vi "Xml_Create_Default.vi"(8 "error in (no error)":errorcluster) -> (0 "error out":errorcluster)   [LabVIEW 2018]
doc: "This example demonstrates how to convert a LabVIEW data structure into an XML string using the GXML reference library."
uses:
  controls/TRAPPING_Inputs.ctl
  controls/SPECTRUM.ctl
  controls/VOLTAGES_Inputs.ctl
  controls/HEXA_Inputs.ctl
  controls/QUAD_Inputs.ctl
  controls/DATA_Inputs.ctl
  controls/PROCESSING_Inputs.ctl
  controls/HARDWARE_Inputs.ctl
  controls/AO_6711_Inputs.ctl
  controls/AWG_5421_Inputs.ctl
  <instrlib>/niFgen/niFgen.llb/niFgen_ctl Trigger Source Values (Ring).ctl
  controls/DIGIT_5122_Inputs.ctl
  <instrlib>/niScope/Controls/niScope trigger source.ctl
  controls/HSDIO_6541_Inputs.ctl
  <instrlib>/niHSDIO/niHSDIO.llb/niHSDIO_ctl Trigger Source Values (Ring).ctl
  controls/EXPERT_Inputs.ctl
  controls/SOFTWARE_Inputs.ctl
  controls/XML_Inputs.ctl
  controls/TIMING_Inputs.ctl
  controls/EXCIT_Table.ctl
  controls/EXCIT_Inputs.ctl
  controls/EXPERT_Path_Selector.ctl
  <vilib>/NI/GXML/GXML.lvlib
panel:
  out "chemin complet":path
  in  "EXCIT Table":T1={"Number of Excits"=0, "Number of Ejects"=0, "Sampling Frequency"=0.0, "Waveforms Table"=[["Excit1", "name", "Swift", "0.5", "1200", "70", "150", "550", "0", "0", "0"]]}
  in  "SOFTWARE Inputs":T2={"Application Directory"=path "D:/S.O.F.T.S/LABVIEW/PIL", "Software Version"="1.0.0", "Data Path"=path "D:/PIRENEA/DATA", "XML Path"=path "D:/PIRENEA/DATA", "XML File Filter"="*.xml", "XML Saved Path"=path "D:/PIRENEA/SAVED_XML", "Excit Scripts Path"=path "D:/PIRENEA/TECHNICAL/EXCIT_SCRIPTS", "Excit Scripts File Filter"="*.txt", "Excit Waveforms Path"=path "D:/PIRENEA/TECHNICAL/EXCIT_WFMS", "Excit Waveforms File Filter"="*.bin", "Timing Scripts Path"=path "D:/PIRENEA/TECHNICAL/TIMING_SCRIPTS", "Timing Scripts File Filter"="*.txt", "Timing Waveforms Path"=path "D:/PIRENEA/TECHNICAL/TIMING_WFMS", "Timing Waveforms File Filter"="*.bin", "Trapping Waveforms Path"=path "D:/PIRENEA/TECHNICAL/TRAPPING_WFMS", "Trapping Waveforms File Filter"="*.bin"}
  in  "TIMING Inputs":T3={"Number of Acquisitions "=1, "Number of Accumulations"=1, "Table of Waveforms"=[], "Script Text"=""} caption="SEQUENCE Inputs" {"Number of Accumulations" min=0 max=50 step=1; "Number of Acquisitions" min=1 max=10 step=1}
  in  "EXPERT Inputs":T4={"DIGIT 5122 Inputs"={"Sample Rate"=10000.0, "Resource Name"="DIGIT_5122", "Channel Name"="0", "Trigger Source"="VAL_EXTERNAL", "Vertical Range"=10.0, "Trigger Level"=3.0}, "HSDIO 6541 Inputs"={"Resource Name"="HSDIO_6541", "Clock Rate"=1000000.0, "Trigger Source"="PFI0"}, "SOFTWARE Inputs"={"Application Directory"=path "D:/S.O.F.T.S/LABVIEW/PIL", "Software Version"="1.0.0", "Data Path"=path "D:/PIRENEA/DATA", "XML Path"=path "D:/PIRENEA/DATA", "XML File Filter"="*.xml", "XML Saved Path"=path "D:/PIRENEA/DATA", "Excit Scripts Path"=path "D:/PIRENEA/EXCIT_SCRIPTS", "Excit Scripts File Filter"="*.txt", "Excit Waveforms Path"=path "D:/PIRENEA/EXCIT_WFMS", "Excit Waveforms File Filter"="*.bin", "Timing Scripts Path"=path "D:/PIRENEA/SEQUENCE_SCRIPTS", "Timing Scripts File Filter"="*.txt", "Timing Waveforms Path"=path "D:/PIRENEA/SEQUENCE_WFMS", "Timing Waveforms File Filter"="*.bin", "Trapping Waveforms Path"=path "D:/PIRENEA/TRAPPING_WFMS", "Trapping Waveforms File Filter"="*.bin"}, "AO 6711 Inputs"={"Physical Channels"="AO_6711/ao0:3", "Min Voltage"=-10.0, "Max Voltage"=10.0, "Trigger Source"="/AO_6711/PFI0", "Counter"="AO_6711/ctr0"}, "AWG 5421 Inputs"={"Resource Name"="AWG_5421", "Sample Rate"=20000000.0, "Trigger Type"=2, "Trigger Source"="PFI0", "Waveform Gain"=0.31, "Digital Filter ON"=TRUE}, "XML Inputs"={"Version Tag Name"="XML_Version", "Version String"="1.0"}} {"AWG 5421 Inputs"."Sample Rate" format="%.2p"; "AWG 5421 Inputs"."Trigger Type" items=["None", "Software Edge", "Digital Edge", "Digital Level"]; "AO 6711 Inputs"."Max Voltage" min=-10.0 max=10.0; "AO 6711 Inputs"."Min Voltage" min=-10.0 max=10.0; "HSDIO 6541 Inputs"."Clock Rate" format="%.2p"; "DIGIT 5122 Inputs"."Trigger Level" format="%.2f"; "DIGIT 5122 Inputs"."Vertical Range" format="%.2f"; "DIGIT 5122 Inputs"."Sample Rate" step=65535.0 format="%#_3p"}
  in  "HARDWARE Inputs":T13={"AO 6711 Inputs"={"Physical Channels"="AO_6711/ao0:3", "Min Voltage"=-10.0, "Max Voltage"=10.0, "Trigger Source"="/AO_6711/PFI3", "Counter"="AO_6711/ctr0"}, "AWG 5421 Inputs"={"Resource Name"="AWG_5421", "Sample Rate"=10000000.0, "Trigger Type"=2, "Trigger Source"="PFI0", "Waveform Gain"=0.31, "Digital Filter ON"=TRUE}, "DIGIT 5122 Inputs"={"Sample Rate"=10000.0, "Resource Name"="DIGIT_5122", "Channel Name"="0", "Trigger Source"="VAL_EXTERNAL", "Vertical Range"=10.0, "Trigger Level"=3.0}, "HSDIO 6541 Inputs"={"Resource Name"="HSDIO_6541", "Clock Rate"=1000000.0, "Trigger Source"="PFI0"}} {"HSDIO 6541 Inputs"."Clock Rate" format="%.2p"; "DIGIT 5122 Inputs"."Trigger Level" format="%.2f"; "DIGIT 5122 Inputs"."Vertical Range" format="%.2f"; "DIGIT 5122 Inputs"."Sample Rate" step=65535.0 format="%#_3p"; "AWG 5421 Inputs"."Sample Rate" format="%.2p"; "AWG 5421 Inputs"."Trigger Type" items=["None", "Software Edge", "Digital Edge", "Digital Level"]; "AO 6711 Inputs"."Max Voltage" min=-10.0 max=10.0; "AO 6711 Inputs"."Min Voltage" min=-10.0 max=10.0}
  in  "PROCESSING Inputs":T14={"Reference Mass"=300.0939, "Cyclotron Freq"=255.727, "Magnetron Freq"=0.001} {"Magnetron Freq" format="%.5g"; "Cyclotron Freq" format="%.5g"; "Reference Mass" format="%.5g"}
  in  "DATA Inputs":T15={"Record Length"=100000, "Sample Rate"=10000000.0, "Data Type"=0, "Vertical Range"=0.4, "Acquisition Duration"=100000.0} {"Vertical Range" items=["0.2"=0.2, "0.4"=0.4, "1"=1.0, "2"=2.0, "4"=4.0, "10"=10.0]; "Data Type" items=["I16", "DBL"]; "Sample Rate" items=["1 MHz"=1000000.0, "2 MHz"=2000000.0, "5 MHz"=5000000.0, "10 MHz"=10000000.0, "20 MHz"=20000000.0, "25 MHz"=25000000.0, "50 MHz"=50000000.0, "100 MHz"=100000000.0]}
  in  "Version String":string="1.4"
  in  "Version Tag Name":string="XML_Version"
  out "Version String":string
  in  "VOLTAGES Inputs":T16={"Hexa 1"={"Used"=TRUE, "Voltage"=0.1}, "Hexa 2"={"Used"=TRUE, "Voltage"=0.2}, "Hexa 3"={"Used"=TRUE, "Voltage"=0.3}, "Quad 1"={"Used"=TRUE, "Voltage"=1.1}, "Quad 2"={"Used"=TRUE, "Voltage"=1.2}, "Quad 3"={"Used"=TRUE, "Voltage"=1.3}}
  in  "SPECTRUM":T19={"Day Path"=path "D:/PIRENEA/DATA/2016/data_2016_01_01", "Spectrum Name"="2016_01_01_000.A00", "Accumulated"=FALSE, "Stored in Database"=FALSE, "From a Set of"=1, "Quality Flag"="Optimal"}
  in  "TRAPPING Inputs":T20={"Number of Channels"=4, "Init Values"=[2.0, 9.0, 2.0, 9.0], "Opening Values"=[0.0, 0.0, 0.0, 0.0], "Trapping Values"=[2.0, 9.0, 2.0, 9.0], "Emptying Values"=[-10.0, -10.0, -10.0, -10.0], "Adiabatic ON"=FALSE, "Adiabatic Duration"=0, "Adiabatic Waveforms"=["Adiabatic_None_2_2_2000", "Adiabatic_Ramp_9_0_2000", "Adiabatic_DoubleRamp_2_0_2000", "Adiabatic_RC_9_0_2000"], "Ions Accumulation ON"=FALSE, "Number of Ions Refills"=1, "Ions Opening Values"=[0.0, 0.0, 0.0, 0.0], "Ions Trapping Values"=[2.0, 9.0, 2.0, 9.0]} {"Number of Ions Refills" min=1 max=1000; "Ions Opening Values" min=-10.0 max=10.0; "Ions Trapping Values" min=-10.0 max=10.0; "Trapping Values" min=-10.0 max=10.0; "Init Values" min=-10.0 max=10.0; "Emptying Values" min=-10.0 max=10.0; "Opening Values" min=-10.0 max=10.0}
  in  "Save XML to File?":bool
  out "Concatenated GXML String":string
  # "HEXAPOLE"
  # "QUADRIPOLE"
  # "GO_out"
  # "Gout"
  # "GI_in"
  # "Gin"
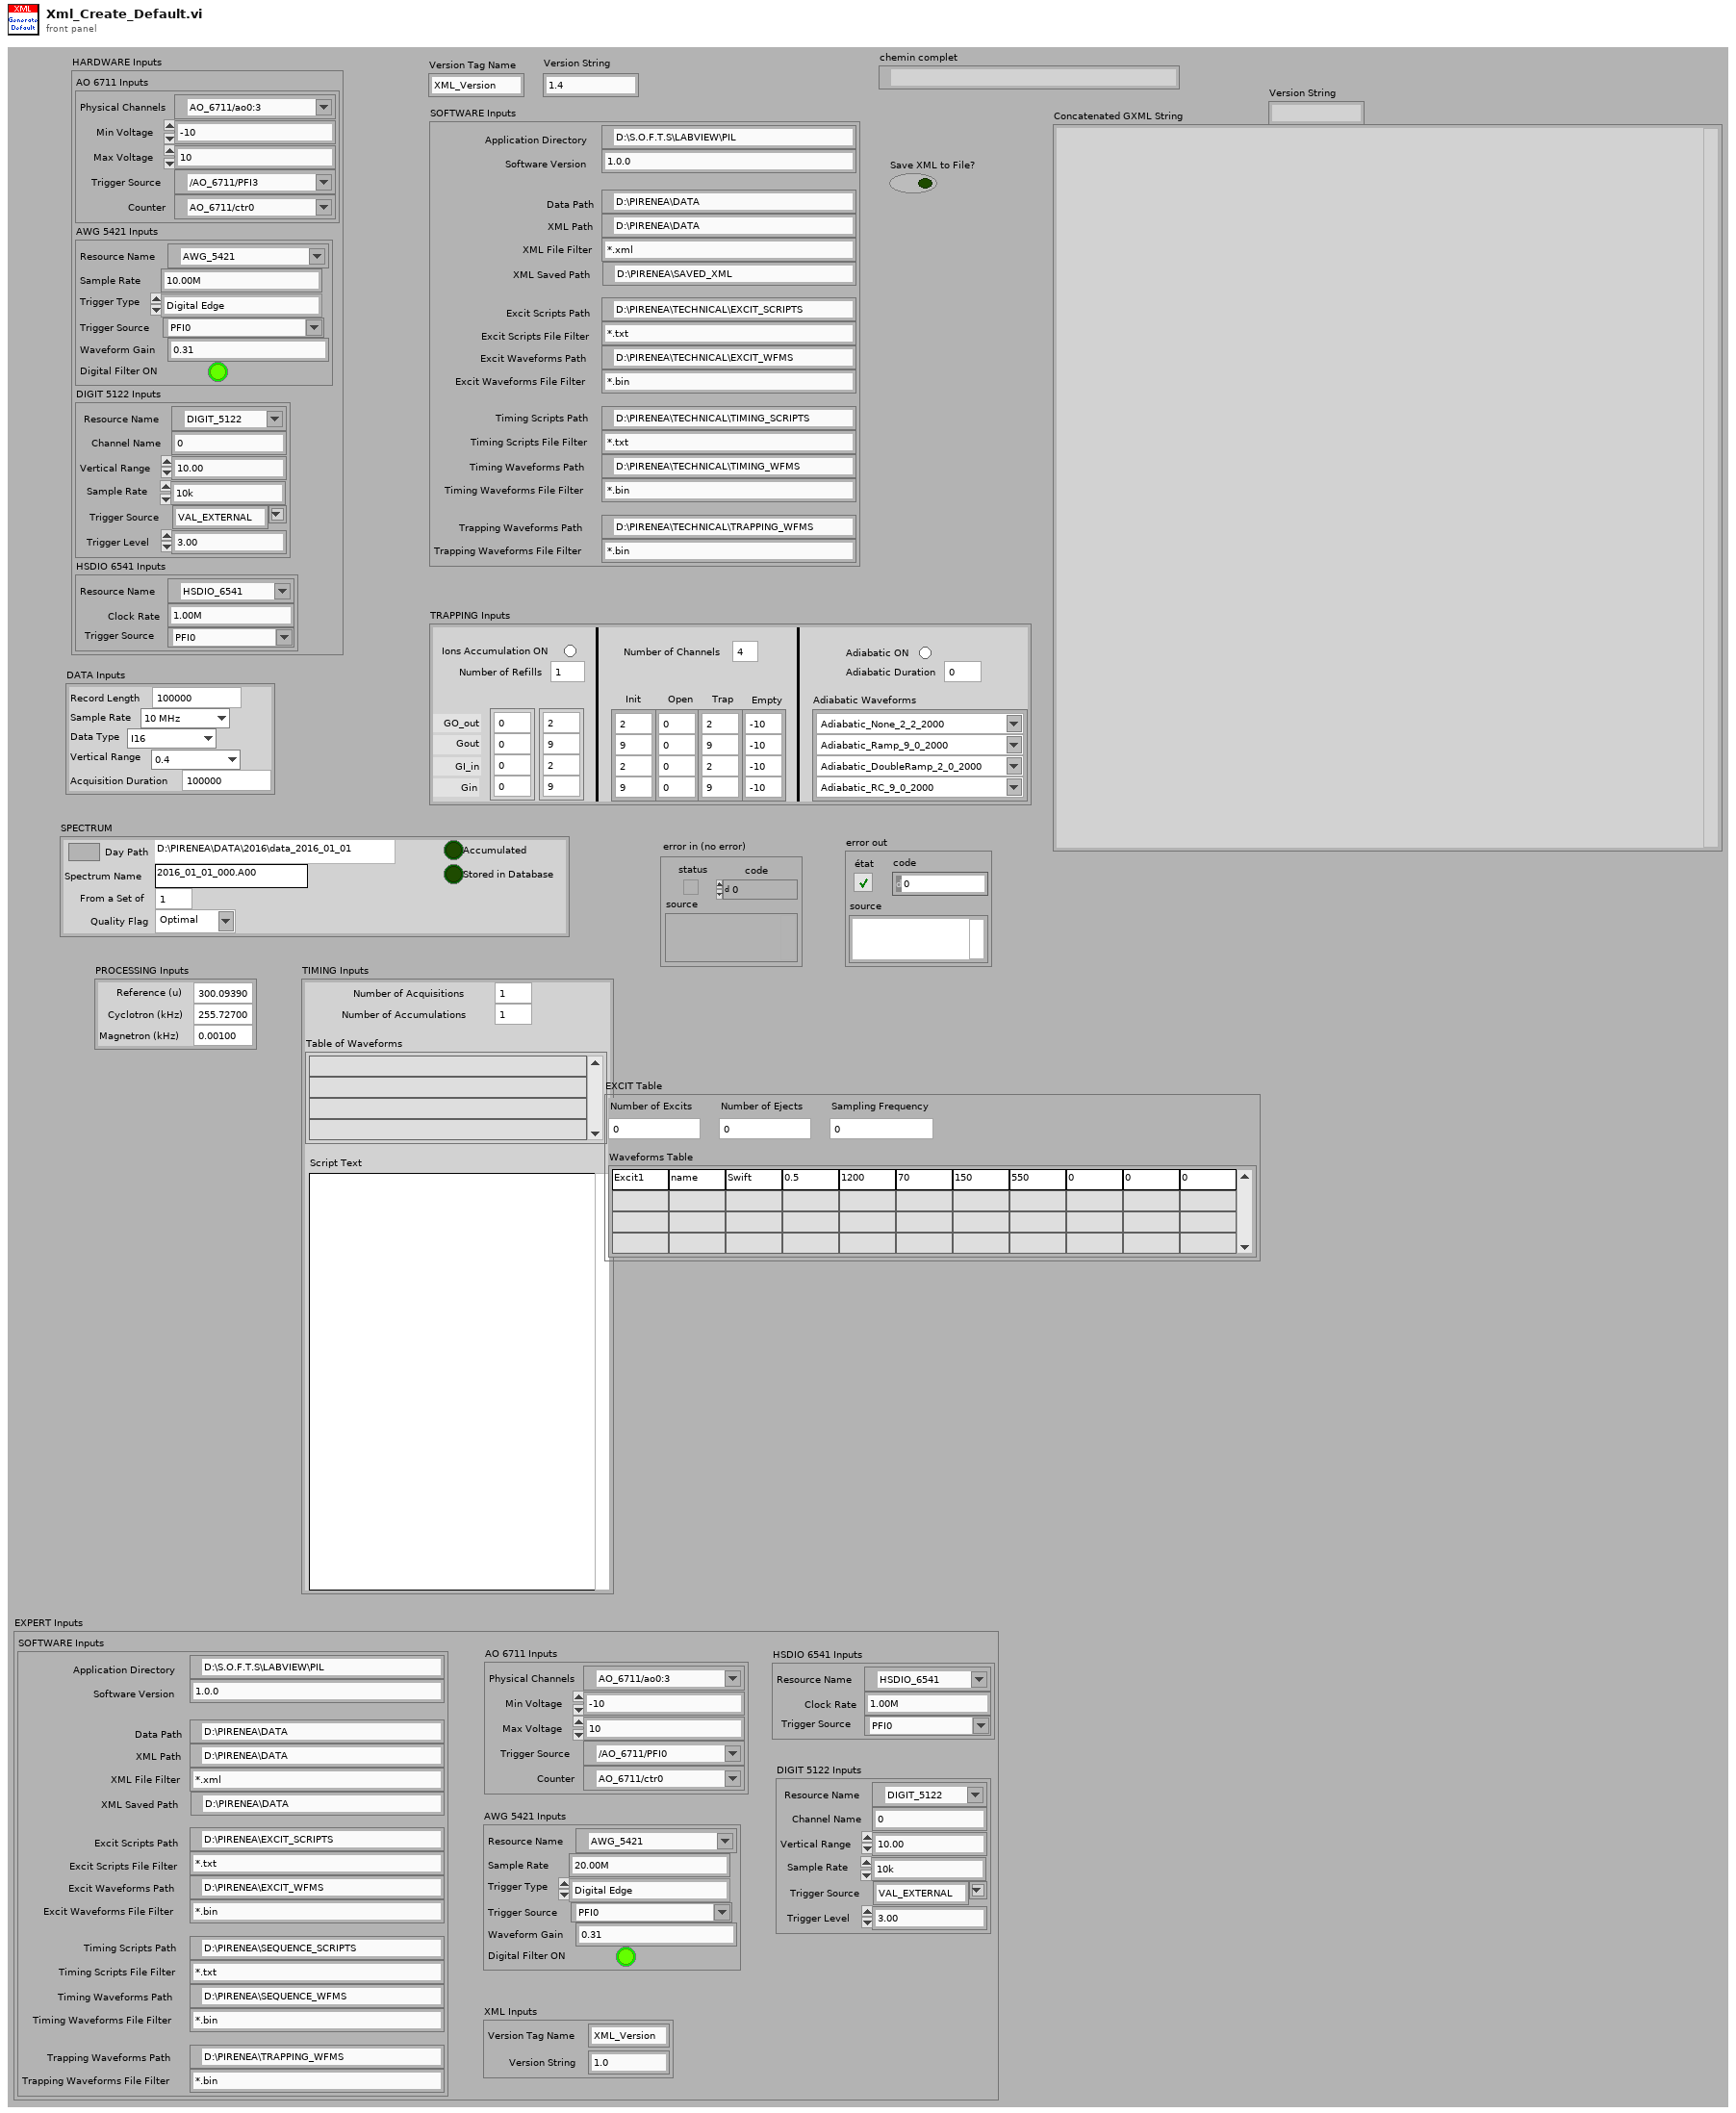
[diagram p1: front panel]
types:
  T1 = typedef "EXCIT_Table.ctl" = cluster{"Number of Excits":u16, "Number of Ejects":u16, "Sampling Frequency":dbl, "Waveforms Table":string[][]}
  T2 = typedef "SOFTWARE_Inputs.ctl" = cluster{"Application Directory":path, "Software Version":string, "Data Path":path, "XML Path":path, "XML File Filter":string, "XML Saved Path":path, "Excit Scripts Path":path, "Excit Scripts File Filter":string, "Excit Waveforms Path":path, "Excit Waveforms File Filter":string, "Timing Scripts Path":path, "Timing Scripts File Filter":string, "Timing Waveforms Path":path, "Timing Waveforms File Filter":string, "Trapping Waveforms Path":path, "Trapping Waveforms File Filter":string}
  T3 = typedef "TIMING_Inputs.ctl" = cluster{"Number of Acquisitions ":i16, "Number of Accumulations":i16, "Table of Waveforms":string[], "Script Text":string}
  T4 = typedef "EXPERT_Inputs.ctl" = cluster{"DIGIT 5122 Inputs":T5, "HSDIO 6541 Inputs":T7, "SOFTWARE Inputs":T2, "AO 6711 Inputs":T9, "AWG 5421 Inputs":T10, "XML Inputs":T12}
  T5 = typedef "DIGIT_5122_Inputs.ctl" = cluster{"Sample Rate":dbl, "Resource Name":refnum<k15>, "Channel Name":string, "Trigger Source":T6, "Vertical Range":dbl, "Trigger Level":dbl}
  T6 = typedef "niScope trigger source.ctl" = string
  T7 = typedef "HSDIO_6541_Inputs.ctl" = cluster{"Resource Name":refnum<k15>, "Clock Rate":dbl, "Trigger Source":T8}
  T8 = typedef "niHSDIO_ctl Trigger Source Values (Ring).ctl" = string
  T9 = typedef "AO_6711_Inputs.ctl" = cluster{"Physical Channels":tag, "Min Voltage":dbl, "Max Voltage":dbl, "Trigger Source":tag, "Counter":tag}
  T10 = typedef "AWG_5421_Inputs.ctl" = cluster{"Resource Name":refnum<k15>, "Sample Rate":dbl, "Trigger Type":u16, "Trigger Source":T11, "Waveform Gain":dbl, "Digital Filter ON":bool}
  T11 = typedef "niFgen_ctl Trigger Source Values (Ring).ctl" = string
  T12 = typedef "XML_Inputs.ctl" = cluster{"Version Tag Name":string, "Version String":string}
  T13 = typedef "HARDWARE_Inputs.ctl" = cluster{"AO 6711 Inputs":T9, "AWG 5421 Inputs":T10, "DIGIT 5122 Inputs":T5, "HSDIO 6541 Inputs":T7}
  T14 = typedef "PROCESSING_Inputs.ctl" = cluster{"Reference Mass":dbl, "Cyclotron Freq":dbl, "Magnetron Freq":dbl}
  T15 = typedef "DATA_Inputs.ctl" = cluster{"Record Length":i32, "Sample Rate":dbl, "Data Type":u8, "Vertical Range":dbl, "Acquisition Duration":dbl}
  T16 = typedef "VOLTAGES_Inputs.ctl" = cluster{"Hexa 1":T17, "Hexa 2":T17, "Hexa 3":T17, "Quad 1":T18, "Quad 2":T18, "Quad 3":T18}
  T17 = typedef "HEXA_Inputs.ctl" = cluster{"Used":bool, "Voltage":dbl}
  T18 = typedef "QUAD_Inputs.ctl" = cluster{"Used":bool, "Voltage":dbl}
  T19 = typedef "SPECTRUM.ctl" = cluster{"Day Path":path, "Spectrum Name":string, "Accumulated":bool, "Stored in Database":bool, "From a Set of":i16, "Quality Flag":string}
  T20 = typedef "TRAPPING_Inputs.ctl" = cluster{"Number of Channels":i32, "Init Values":dbl[], "Opening Values":dbl[], "Trapping Values":dbl[], "Emptying Values":dbl[], "Adiabatic ON":bool, "Adiabatic Duration":i32, "Adiabatic Waveforms":string[], "Ions Accumulation ON":bool, "Number of Ions Refills":i32, "Ions Opening Values":dbl[], "Ions Trapping Values":dbl[]}
  T21 = typedef "EXPERT_Path_Selector.ctl" = enum16{"Application", "Resources", "Data", "XML", "XML Saved", "Load Directory"}
  T22 = typedef "EXCIT_Inputs.ctl" = cluster{"Number of Excitations":i32, "Script Text":string, "Table of Waveforms":string[]}
  T23 = typedef "EXPERIMENT_Inputs.ctl" = cluster{"Setup":string, "Date":string, "User Name":string, "Comment":string, "Experiment Procedures":string[], "Chemical Source":string, "Sample Components":string[], "Species":string[], "Laser 1":T24, "Laser 2":T24, "Laser 3":T24, "Laser 4":T24, "Laser 5":T24, "Lamp 1":T25, "Lamp 2":T25, "Gas 1":T26, "Gas 2":T26, "Gas 3":T26, "Gas 4":T26, "Gas 5":T26}
  T24 = typedef "LASER_Inputs.ctl" = cluster{"Used":bool, "Name":string, "Wavelength":dbl, "Energy":dbl}
  T25 = typedef "LAMP_Inputs.ctl" = cluster{"Used":bool, "Name":string, "Wavelength":dbl, "Attenuation":dbl}
  T26 = typedef "GAS_Inputs.ctl" = cluster{"Used":bool, "Name":string, "Pressure":dbl}
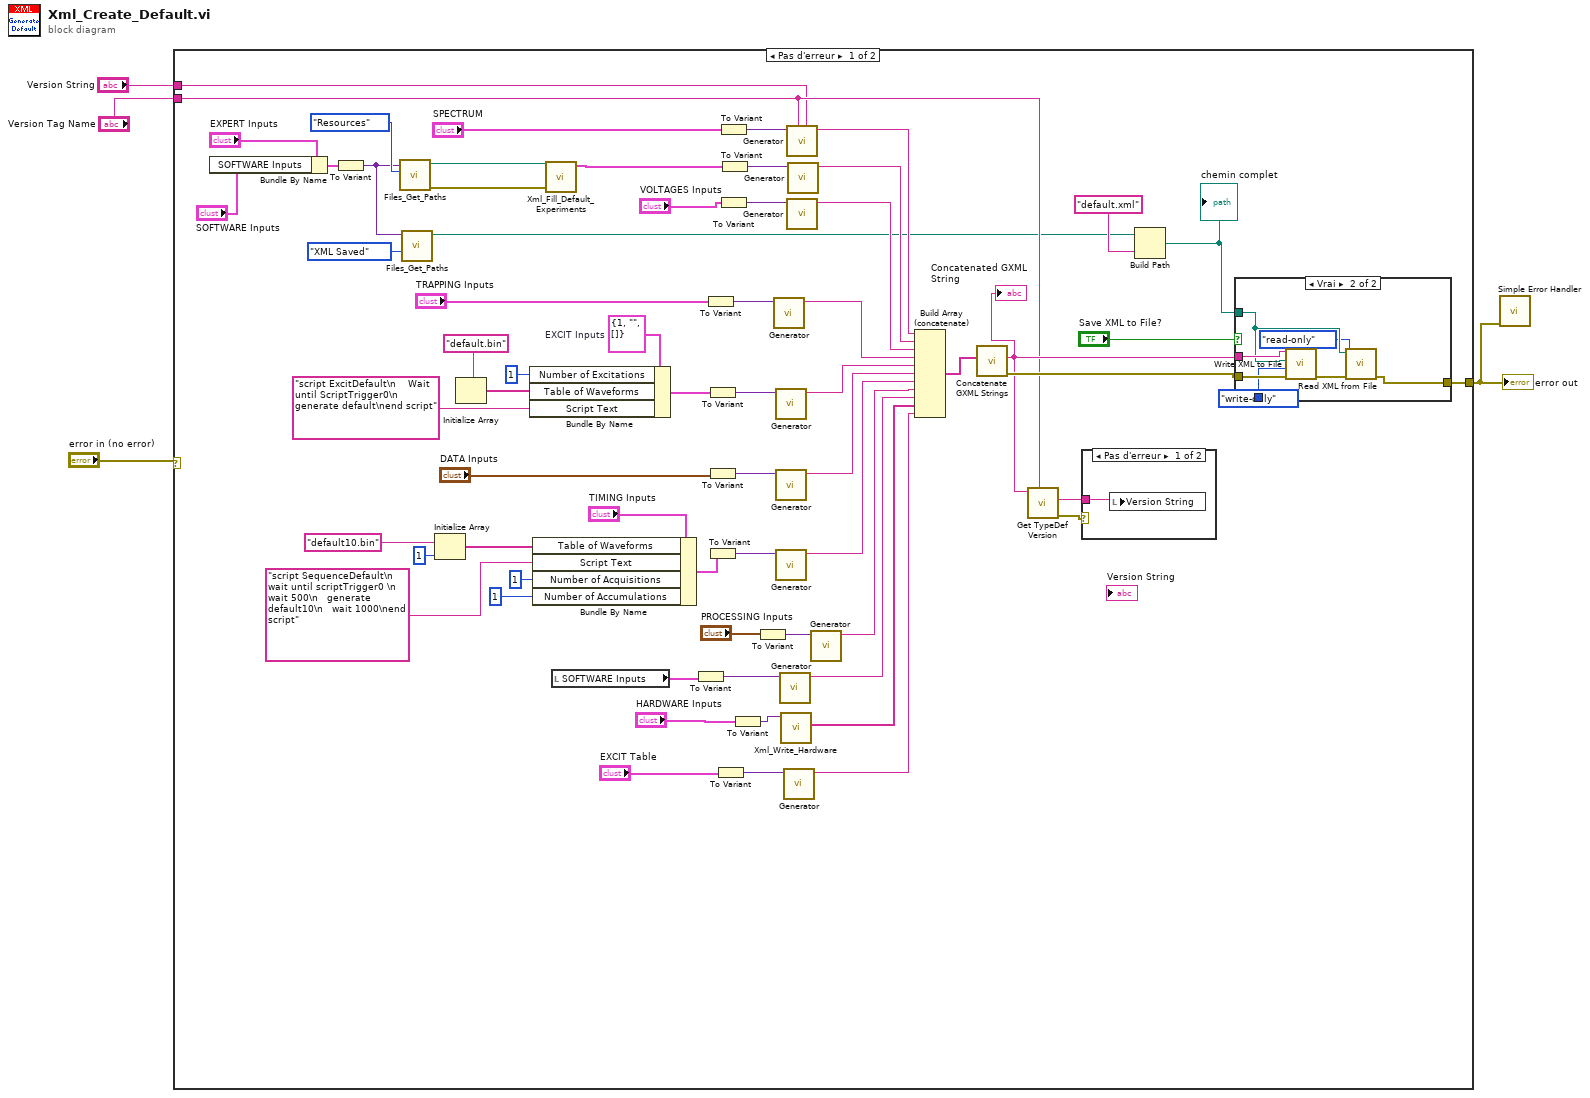
[diagram p0: block diagram]
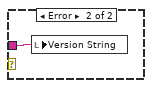
[diagram p2: hidden frame]
diagram:
  n1 = case shown="Pas d'erreur" "error in (no error)" {
    selector: "error in (no error)" -> [_ w81]
    tunnel: [w66 w81] -> w3
    tunnel: "Version String" -> [w26 _]
    tunnel: "Version Tag Name" -> [w27 _]
    frame No Error {
      w62 = T22 {"Number of Excitations"=1, "Script Text"="", "Table of Waveforms"=[]}  # EXCIT Inputs
      n2 = Bundle By Name(cluster="EXPERT Inputs", "SOFTWARE Inputs"="SOFTWARE Inputs") -> (w18:T4)
      n3 = To Variant(anything=w18) -> (Variant=w8:variant)
      n4 = call "Files_Get_Paths.vi"("EXPERT Path Selector"=EXPERT_Path_Selector."Resources", "Variant"=w8) -> ("error out"=w14:errorcluster, "Path"=w12:path)  [unwired: 8 in]
      n5 = call "Files_Get_Paths.vi"("EXPERT Path Selector"=EXPERT_Path_Selector."XML Saved", "Variant"=w8) -> ("Path"=w6:path)  [unwired: 8 in, 1 out]
      n6 = Initialize Array("default10.bin" ("élément"), 1 ("taille de la dimension")) -> (w52:string[])
      n7 = Initialize Array("default.bin" ("élément")) -> (w59:string[])  [unwired: 1 in]
      n8 = Bundle By Name(cluster=w62, "Number of Excitations"=1, "Table of Waveforms"=w59, "Script Text"="script ExcitDefault\n    Wait until ScriptTrigger0\n    generate default\nend script" ("Script text")) -> (w56:T22)
      n9 = Bundle By Name(cluster="TIMING Inputs", "Table of Waveforms"=w52, "Script Text"="script SequenceDefault\n   wait until scriptTrigger0 \n   wait 500\n   generate default10\n   wait 1000\nend script" ("Script text"), "Number of Acquisitions"=i16 1 ("Number Of Acquisitions"), "Number of Accumulations"=i16 1 ("Number Of Accumulations")) -> (w49:T3)
      n10 = call "Xml_Fill_Default_Experiments.vi"("error in (no error)"=w14, "Resources Path"=w12) -> ("EXPERIMENT Inputs"=w44:T23)  [unwired: 6 in, 1 out]
      n11 = local read "SOFTWARE Inputs"() -> (w13:T2)
      n12 = To Variant(anything=w13) -> (Variant=w69:variant)
      n13 = To Variant(anything="TRAPPING Inputs") -> (Variant=w64:variant)
      n14 = To Variant(anything=w56) -> (Variant=w57:variant)
      n15 = To Variant(anything="DATA Inputs") -> (Variant=w55:variant)
      n16 = To Variant(anything=w49) -> (Variant=w50:variant)
      n17 = To Variant(anything="EXCIT Table") -> (Variant=w11:variant)
      n18 = To Variant(anything="SPECTRUM") -> (Variant=w47:variant)
      n19 = To Variant(anything="VOLTAGES Inputs") -> (Variant=w39:variant)
      n20 = To Variant(anything=w44) -> (Variant=w70:variant)
      n21 = To Variant(anything="HARDWARE Inputs") -> (Variant=w36:variant)
      n22 = To Variant(anything="PROCESSING Inputs") -> (Variant=w23:variant)
      n23 = call <vilib>:"Generator.vi"("Variant"=w64) -> ("XML String Out"=w31:string)  [unwired: 9 in, 1 out]
      n24 = call <vilib>:"Generator.vi"("Variant"=w57) -> ("XML String Out"=w32:string)  [unwired: 9 in, 1 out]
      n25 = call <vilib>:"Generator.vi"("Variant"=w55) -> ("XML String Out"=w33:string)  [unwired: 9 in, 1 out]
      n26 = call <vilib>:"Generator.vi"("Variant"=w50) -> ("XML String Out"=w34:string)  [unwired: 9 in, 1 out]
      n27 = call <vilib>:"Generator.vi"("Variant"=w69) -> ("XML String Out"=w35:string)  [unwired: 9 in, 1 out]
      n28 = call "Xml_Write_Hardware.vi"("Variant"=w36) -> ("XML String Out"=w21:string[])  [unwired: 8 in, 2 out]
      n29 = call <vilib>:"Generator.vi"("Variant"=w11) -> ("XML String Out"=w9:string)  [unwired: 9 in, 1 out]
      n30 = call <vilib>:"Generator.vi"("Version String"=w26, "Version Tag Name"=w27, "Variant"=w47) -> ("XML String Out"=w41:string)  [unwired: 7 in, 1 out]
      n31 = call <vilib>:"Generator.vi"("Variant"=w39) -> ("XML String Out"=w37:string)  [unwired: 9 in, 1 out]
      n32 = call <vilib>:"Generator.vi"("Variant"=w70) -> ("XML String Out"=w40:string)  [unwired: 9 in, 1 out]
      n33 = call <vilib>:"Generator.vi"("Variant"=w23) -> ("XML String Out"=w19:string)  [unwired: 9 in, 1 out]
      n34 = Build Array (concatenate)(w41, w40, w37, w31, w32, w33, w34, w19, w35, w21, w9) -> (w68:string[])
      n35 = call <vilib>:"Concatenate GXML Strings.vi"("GXML Strings"=w68) -> ("error out"=w67:errorcluster, "Concatenated GXML String"=w30:string)  [unwired: 9 in]
      "Concatenated GXML String" <- w30
      n36 = call <vilib>:"Get TypeDef Version.vi"("Version Tag Name"=w27, "XML String In"=w30) -> ("error out"=w28:errorcluster, "Version String"=w29:string)  [unwired: 7 in, 1 out]
      n37 = case shown="Pas d'erreur" w28 {
        tunnel: w29 -> [w71 w72]
        frame No Error {
          n38 = local write "Version String"(w71) -> ()
        }
        frame Error {
          n39 = local write "Version String"(w72) -> ()
        }
      }
      n40 = Build Path(base path=w6, name or relative path="default.xml" ("nom ou chemin relatif")) -> (appended path=w20:path)
      "chemin complet" <- w20
      n41 = case shown="Vrai" "Save XML to File?" {
        tunnel: [w73 w76] -> w66
        tunnel: w30 -> [_ w80]
        tunnel: w67 -> [w73 w79]
        tunnel: w20 -> [_ w77]
        tunnel: enum16{"read/write", "read-only", "write-only"}."write-only" ("file access") -> [_ w75]
        frame False {
        }
        frame True {
          n42 = call <vilib>:"Write XML to File.vi"("error in"=w79, "file access"=w75, "XML File Path"=w77, "XML Input"=w80) -> ("error out"=w78:errorcluster)  [unwired: 7 in]
          n43 = call <vilib>:"Read XML from File.vi"("error in"=w78, "file access"=enum16{"read/write", "read-only", "write-only"}."read-only", "XML File Path"=w77) -> ("error out"=w76:errorcluster)  [unwired: 7 in, 1 out]
        }
      }
    }
    frame Error {
    }
  }
  "error out" <- w3
  n44 = call <vilib>:"Simple Error Handler.vi"("error in (no error)"=w3) -> ()  [unwired: 4 in, 5 out]
